vi "UI_test.vi"() -> ()   [LabVIEW 2017]
panel:
  out "appended array":u8[](array[numeric])
  out "*(type *) &x 2":u32
  out "32bit integer":i32
  out "(hi.lo)":u32
  out "*(type *) &x":sgl format="%.10f"
  out "number":u32
  out "Numeric":dbl
  out "double precision float":dbl
  out "Output_SGL":sgl=92.92 format="%.10f"
  out "Exponent":i32=6
  out "Mantissa":bool[](array[boolean])=[FALSE, TRUE, TRUE, TRUE, FALSE, FALSE, TRUE, TRUE, TRUE, FALSE, TRUE, FALSE, TRUE, TRUE, TRUE, FALSE, FALSE, FALSE, FALSE, TRUE, FALSE, TRUE, FALSE]
  out "Exponent 2":bool[](array[boolean])=[TRUE, FALSE, FALSE, FALSE, FALSE, TRUE, FALSE, TRUE]
  out "Sign":bool
  out "Mantissa 2":dbl=1.4518749713897705 format="%.8f"
  in  "Input_U8":u8[](array[numeric])
  out "appended array 1D":bool[](array[boolean])
  in  "stop":bool
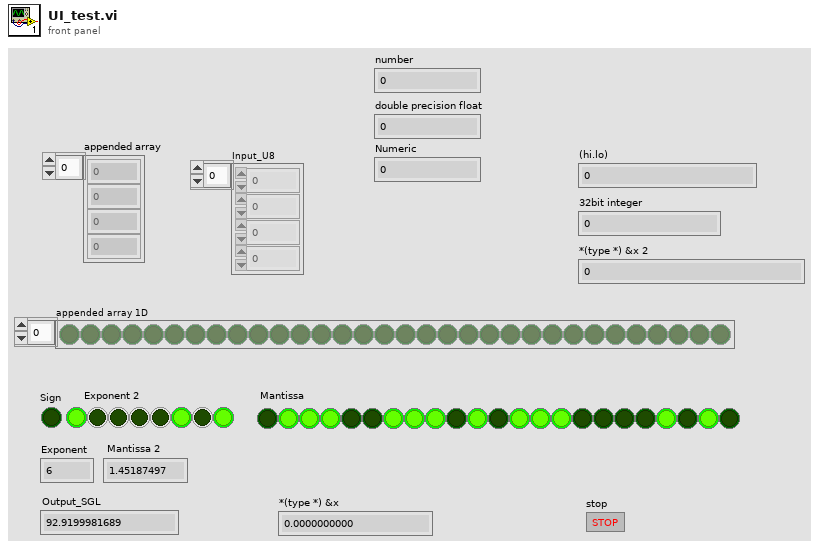
[diagram p1: front panel]
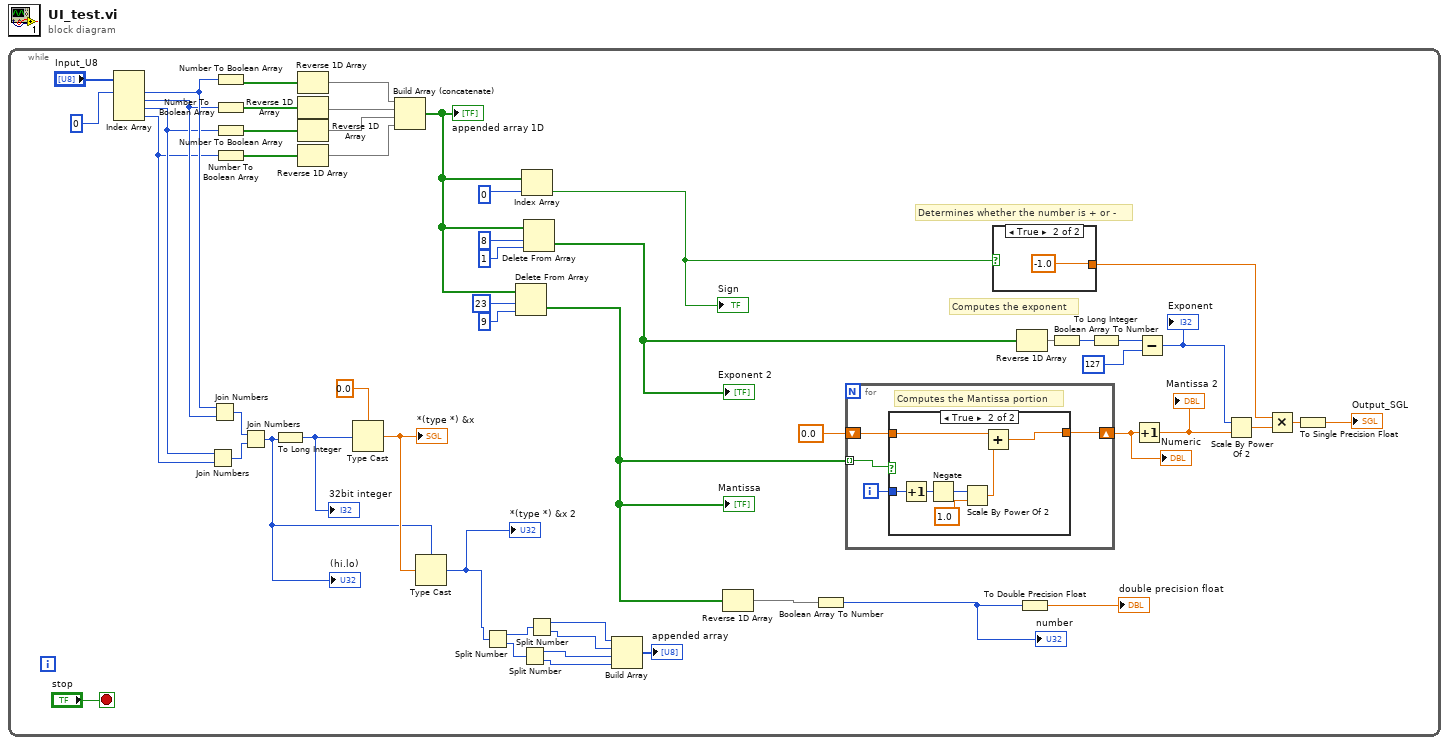
[diagram p0: block diagram]
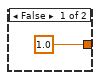
[diagram p2: hidden frame]
diagram:
  n1 = while {
    stop <- "stop" stop-if-true
    # "Computes the exponent"
    # "Determines whether the number is + or -"
    n2 = Index Array(array="Input_U8", index #1=0 ("index")) -> (element #1=w21:u8, element #2=w20:u8, element #3=w19:u8, element #4=w18:u8)  [unwired: 3 in]
    n3 = Join Numbers(hi=w19, lo=w18) -> ((hi.lo)=w16:u16)
    n4 = Join Numbers(hi=w21, lo=w20) -> ((hi.lo)=w17:u16)
    n5 = Number To Boolean Array(number=w21) -> (Boolean array=w31:bool[])
    n6 = Number To Boolean Array(number=w20) -> (Boolean array=w30:bool[])
    n7 = Number To Boolean Array(number=w19) -> (Boolean array=w29:bool[])
    n8 = Number To Boolean Array(number=w18) -> (Boolean array=w28:bool[])
    n9 = Join Numbers(hi=w17, lo=w16) -> ((hi.lo)=w9:u32)
    "(hi.lo)" <- w9
    n10 = To Long Integer(number=w9) -> (32bit integer=w11:i32)
    "32bit integer" <- w11
    n11 = Reverse 1D Array(array=w31) -> (reversed array=w32:bool[])
    n12 = Reverse 1D Array(array=w30) -> (reversed array=w25:bool[])
    n13 = Reverse 1D Array(array=w29) -> (reversed array=w26:bool[])
    n14 = Reverse 1D Array(array=w28) -> (reversed array=w27:bool[])
    n15 = Type Cast(type=sgl 0.0 ("double precision float"), x=w11) -> (*(type *) &x=w10:sgl)
    "*(type *) &x" <- w10
    n16 = Build Array (concatenate)(w32, w25, w26, w27) -> (w15:bool[])
    "appended array 1D" <- w15
    n17 = Type Cast(type=w9, x=w10) -> (*(type *) &x=w8:u32)
    "*(type *) &x 2" <- w8
    n18 = Split Number(x=w8) -> (hi(x)=w7:u16, lo(x)=w6:u16)
    n19 = Delete From Array(array=w15, length=23, index=9) -> (deleted portion=w12:bool[])  [unwired: 1 out]
    "Mantissa" <- w12
    n20 = Split Number(x=w6) -> (hi(x)=w3:u8, lo(x)=w2:u8)
    n21 = Index Array(array=w15, index=0) -> (element=w34:bool)
    "Sign" <- w34
    n22 = Delete From Array(array=w15, length=8, index=1) -> (deleted portion=w36:bool[])  [unwired: 1 out]
    "Exponent 2" <- w36
    n23 = Split Number(x=w7) -> (hi(x)=w5:u8, lo(x)=w4:u8)
    n24 = Build Array(w5, w4, w3, w2) -> (→"appended array":u8[])
    n25 = Reverse 1D Array(array=w12) -> (reversed array=w23:bool[])
    n26 = Boolean Array To Number(Boolean array=w23) -> (number=w13:u32)
    "number" <- w13
    n27 = for {
      tunnel: w12 -> [w59] mode=indexing
      shift-right: [w56] -> w51
      shift-left: 0.0 -> [w57]
      i -> [w58]
      # "Computes the Mantissa portion"
      n28 = case shown="True" w59 {
        tunnel: w58 -> [_ w67]
        tunnel: w57 -> [w60 w63]
        tunnel: [w60 w61] -> w56
        frame False {
        }
        frame True {
          n29 = Increment(x=w67) -> (x+1=w66:i32)
          n30 = Negate(x=w66) -> (-x=w65:i32)
          n31 = Scale By Power Of 2(n=w65, x=1.0) -> (x*2^n=w62:dbl)
          n32 = Add(x=w63, y=w62) -> (x+y=w61:dbl)
        }
      }
    }
    "Numeric" <- w51
    n33 = case shown="True" w34 {
      tunnel: [1.0 -1.0] -> w45
      frame False {
      }
      frame True {
      }
    }
    n34 = Reverse 1D Array(array=w36) -> (reversed array=w47:bool[])
    n35 = To Double Precision Float(number=w13) -> (double precision float=→"double precision float":dbl)
    n36 = Boolean Array To Number(Boolean array=w47) -> (number=w43:u32)
    n37 = To Long Integer(number=w43) -> (32bit integer=w42:i32)
    n38 = Increment(x=w51) -> (x+1=w49:dbl)
    "Mantissa 2" <- w49
    n39 = Subtract(x=w42, y=127) -> (x-y=w44:i32)
    "Exponent" <- w44
    n40 = Scale By Power Of 2(n=w44, x=w49) -> (x*2^n=w48:dbl)
    n41 = Multiply(x=w45, y=w48) -> (x*y=w46:dbl)
    n42 = To Single Precision Float(number=w46) -> (single precision float=→"Output_SGL":sgl)
  }
